vi "ContourAuto1010.vi"   [LabVIEW 2013]
uses:
  <vilib>/Heliosphere Research LLC/Advanced Plotting Toolkit/api_plotting/ContourProperties.ctl
  <vilib>/Heliosphere Research LLC/Advanced Plotting Toolkit/properties/Line.ctl
  <vilib>/Heliosphere Research LLC/Advanced Plotting Toolkit/properties/Line_Style.ctl
  <vilib>/Heliosphere Research LLC/Advanced Plotting Toolkit/typedefs/PlotColor.ctl
  <vilib>/Heliosphere Research LLC/Advanced Plotting Toolkit/properties/Display.ctl
  <vilib>/Heliosphere Research LLC/Advanced Plotting Toolkit/api_plotting/Contour_Automatic.vi
  <vilib>/Heliosphere Research LLC/Advanced Plotting Toolkit/Advanced Plotting Toolkit.lvlib
types:
  T1 = typedef "Advanced Plotting Toolkit.lvlib/PlotColor.ctl" = u32
  T2 = typedef "Advanced Plotting Toolkit.lvlib/ContourProperties.ctl" = cluster{"Label Contours":bool, "Line":T3, "Display":T5}
  T3 = typedef "Advanced Plotting Toolkit.lvlib/Line.ctl" = cluster{"Style":T4, "Color":T1, "Width":sgl}
  T4 = typedef "Advanced Plotting Toolkit.lvlib/Line_Style.ctl" = enum16{"Automatic", "Solid", "Dashed", "Dotted", "Dash-dot", "Invisible"}
  T5 = typedef "Advanced Plotting Toolkit.lvlib/Display.ctl" = cluster{"Alpha":dbl, "Z Order":dbl}
  T6 = typedef "Advanced Plotting Toolkit.lvlib/PlotID.ctl" = i32
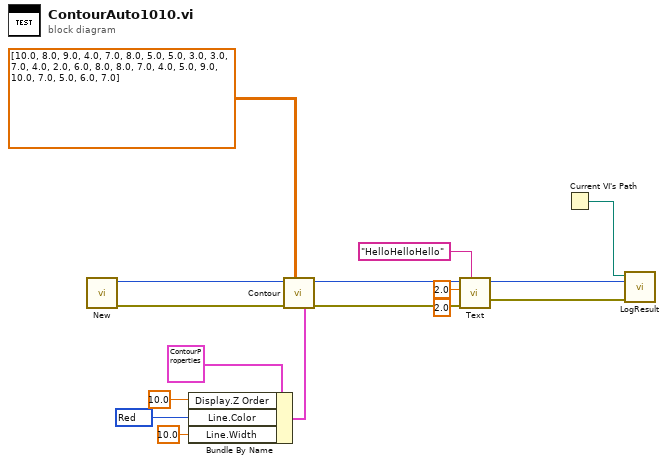
[diagram p0: block diagram]
diagram:
  w9 = T1 16711680 items=["Automatic"=2147483647, "Black"=0, "White"=16777215, "Red"=16711680, "Green"=2263842, "Blue"=255, "Cyan"=65535, "Magenta"=16711935, "Yellow"=16776960] ("Line.Color")
  n1 = call <vilib>:"New.vi"() -> ("error out"=w13:errorcluster, "Plot ID"=w14:T6)  [unwired: 10 in]
  n2 = Bundle By Name(cluster=T2 {"Label Contours"=FALSE, "Line"={"Style"=enum."Automatic", "Color"=2147483647, "Width"=nan}, "Display"={"Alpha"=nan, "Z Order"=nan}} ("Contour Properties"), "Display.Z Order"=sgl 10.0 ("Line.Width"), "Line.Color"=w9, "Line.Width"=sgl 10.0) -> (w11:T2)
  n3 = call-poly <vilib>:"Contour.vi"("Properties"=w11, "Z Data"=dbl[][] [[10.0, 8.0, 9.0, 4.0, 7.0], [8.0, 5.0, 5.0, 3.0, 3.0], [7.0, 4.0, 2.0, 6.0, 8.0], [8.0, 7.0, 4.0, 5.0, 9.0], [10.0, 7.0, 5.0, 6.0, 7.0]], "error in (no error)"=w13, "Plot ID"=w14) -> ("error out"=w4:errorcluster, "Plot ID Out"=w7:T6)  [unwired: 6 in]
  n4 = call <vilib>:"Text.vi"("Text"="HelloHelloHello", "error in (no error)"=w4, "Y Position"=2.0, "X Position"=2.0, "Plot ID"=w7) -> ("error out"=w5:errorcluster, "Plot ID Out"=w6:T6)  [unwired: 5 in]
  n5 = Current VI's Path() -> (path=w16:path)
  n6 = call "LogResult.vi"("Test Result"=w5, "Test Artifact"=w6, "VI Path"=w16) -> ()  [unwired: 9 in]
